vi "qSTE.vi"(0 "System no.":i32=1 min=1 max=4 step=1, 2 "Query axis":string, 5 "error in":errorcluster, 6 "Xo":i32, 7 "N":i32=100, 8 "Nmax":i32=1024) -> (14 "Step response":dbl[](array[numeric]) format="%.6f", 15 "Step size":dbl caption="Numeric" format="%.6f", 19 "error out":errorcluster)   [LabVIEW 2020]
doc: "GCS 1.0 controller: Returns N saved step response points. N must be less than or equal to Nmax. For large N values, communication timeout must be set long enough, otherwise a comm.error may occur.\nGCS 2.0 or higher: Returns STE settings. Use DRR? to read step response points back.\n\nC-843: VI reads step response points. Step size is not valid. Nmax = 32640.\n\nC-843.PM: VI reads step response points. Step size is not valid. Nmax = 32640.\n\nC-848: VI reads step response points. Step size is not valid. Nmax = 1024.\n\nC-866: VI reads step response points. Step size is not valid. Nmax = 32256.\n\nC-880: VI reads step response points. Step size is not valid. Nmax = 1024.\n\nE-517, E-518: VI reads STE settings. Step response is not valid. xo, N and Nmax are not valid.\n\nE-709: VI reads STE settings. Step response is not valid. xo, N and Nmax are not valid.\n\nE-710: VI reads step response points. Step size is not valid. Nmax = 8192.\n\nE-754: VI reads STE settings. Step response is not valid. xo, N and Nmax are not valid.\n\nE-755: VI reads STE settings. Step response, xo, N and Nmax are not valid.\n\nE-761: VI reads step response points. Step size is not valid. Nmax = 8192."
uses:
  Communication/Global1.vi
panel:
  # "GCS 1.0 controller: Returns N saved step response points. N must be \nless than or equal to Nmax. For large N values, communication timeout \nmust be set long enough, otherwise a comm.error may occur.\nGCS 2.0 or higher: Returns STE settings. Use DRR? to read impulse response \npoints back."
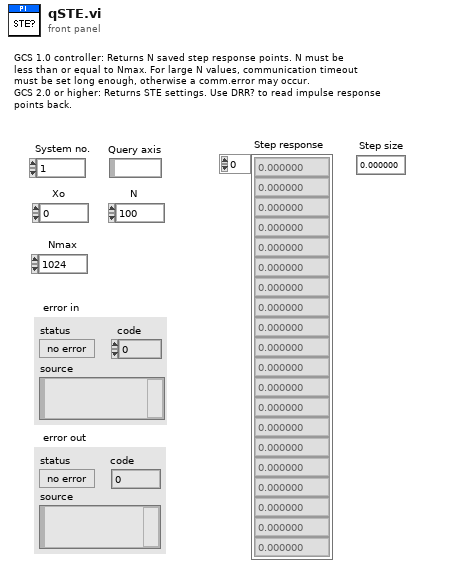
[diagram p1: front panel]
types:
  T1 = typedef "Syntax.ctl" = enum16{"GCS 1.0", "GCS 2.0", "GCS 3.0"}
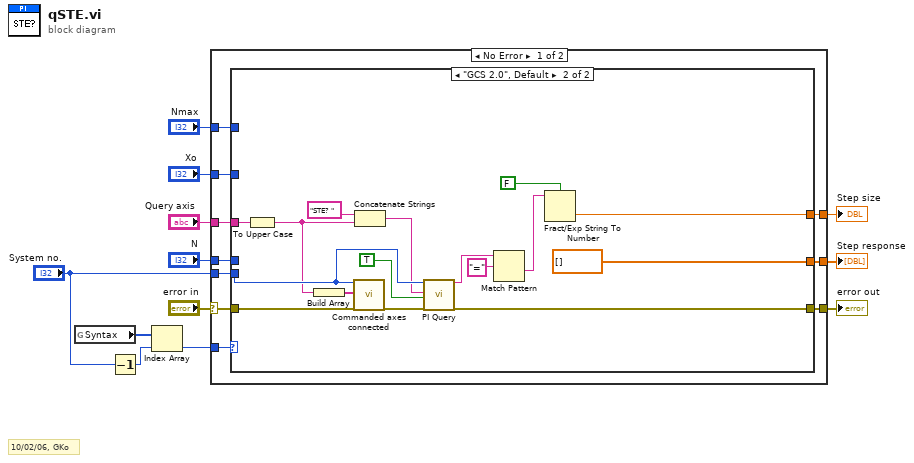
[diagram p0: block diagram]
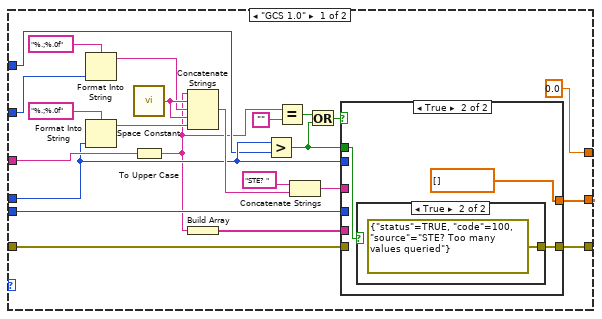
[diagram p2: hidden frame]
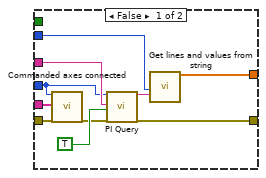
[diagram p3: hidden frame]
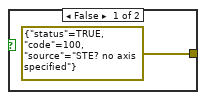
[diagram p4: hidden frame]
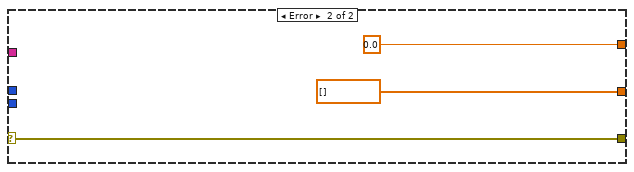
[diagram p5: hidden frame]
diagram:
  # "10/02/06, GKo"
  n1 = global read "Global1.vi" "Syntax"() -> (w5:T1[])
  n2 = Decrement(x="System no.") -> (x-1=w6:i32)
  n3 = Index Array(array=w5, index=w6) -> (element=w1:T1)
  n4 = case shown="No Error" "error in" {
    selector: "error in" -> [w14 w77]
    tunnel: "System no." -> [w22 _]
    tunnel: "Query axis" -> [w21 _]
    tunnel: [w20 w77] -> w11
    tunnel: [w19 dbl[] []] -> w10
    tunnel: "N" -> [w18 _]
    tunnel: "Xo" -> [w17 _]
    tunnel: "Nmax" -> [w16 _]
    tunnel: [w15 0.0] -> w3
    tunnel: w1 -> [w13 _]
    frame No Error {
      n5 = case shown="\"GCS 2.0\", Default" w13 {
        tunnel: w22 -> [w42 w73]
        tunnel: w21 -> [w40 w75]
        tunnel: [w37 w61] -> w20
        tunnel: [w36 dbl[] []] -> w19
        tunnel: w18 -> [w35 _]
        tunnel: w17 -> [w33 _]
        tunnel: w16 -> [w29 _]
        tunnel: w14 -> [w24 w69]
        tunnel: [0.0 w64] -> w15
        frame "GCS 1.0" {
          n6 = Format Into String(format string="%.;%.0f" ("Format String"), w33) -> (resulting string=w31:string)  [unwired: 2 in, 1 out]
          n7 = Format Into String(format string="%.;%.0f" ("Format String"), w35) -> (resulting string=w30:string)  [unwired: 2 in, 1 out]
          n8 = call <vilib>:"Space Constant.vi"() -> ("String"=w32:string)
          n9 = To Upper Case(1:w40) -> (0:w23:string)
          n10 = Concatenate Strings(w23, w32, w31, w32, w30) -> (w38:string)
          n11 = Build Array(w23) -> (w41:string[])
          n12 = Greater?(x=w35, y=w29) -> (0:w25:bool)
          n13 = Equal?(x=w23, y="" ("x")) -> (x = y?=w26:bool)
          n14 = Concatenate Strings("STE? ", w38) -> (w44:string)
          n15 = Or(x=w26, y=w25) -> (x .or. y?=w27:bool)
          n16 = case shown="True" w27 {
            tunnel: w44 -> [w54 _]
            tunnel: w42 -> [w52 _]
            tunnel: w41 -> [w51 _]
            tunnel: w24 -> [w53 _]
            tunnel: [w46 w57] -> w37
            tunnel: w35 -> [w49 _]
            tunnel: [w50 dbl[] [] ("Waveform points")] -> w36
            tunnel: w25 -> [_ w56]
            frame False {
              n17 = call "Commanded axes connected.vi"("System no."=w52, "Commanded axes"=w51, "error in"=w53) -> ("error out"=w48:errorcluster)  [unwired: 1 in, 15 out]
              n18 = call "PI Query.vi"("System no."=w52, "String to send"=w54, "Attach termination char.?"=TRUE ("Attach Linefeed?"), "error in"=w48) -> ("String read"=w47:string, "error out"=w46:errorcluster)  [unwired: 3 in, 11 out]
              n19 = call "Get lines and values from string.vi"("Array size"=w49, "Input string"=w47) -> ("Numerical values"=w50:dbl[])  [unwired: 17 out]
            }
            frame True {
              n20 = case shown="True" w56 {
                tunnel: [errorcluster {"status"=TRUE, "code"=100, "source"="STE? no axis specified"} ("error out") errorcluster {"status"=TRUE, "code"=100, "source"="STE? Too many values queried"} ("error out")] -> w57
                frame False {
                }
                frame True {
                }
              }
            }
          }
        }
        frame "GCS 2.0", Default {
          n21 = To Upper Case(1:w75) -> (0:w68:string)
          n22 = Build Array(w68) -> (w74:string[])
          n23 = call "Commanded axes connected.vi"("System no."=w73, "Commanded axes"=w74, "error in"=w69) -> ("error out"=w70:errorcluster)  [unwired: 1 in, 15 out]
          n24 = Concatenate Strings("STE? ", w68) -> (w71:string)
          n25 = call "PI Query.vi"("System no."=w73, "String to send"=w71, "Attach termination char.?"=TRUE ("Attach Linefeed?"), "error in"=w70) -> ("String read"=w62:string, "error out"=w61:errorcluster)  [unwired: 3 in, 11 out]
          n26 = Match Pattern(string=w62, regular expression="=") -> (after substring=w63:string)  [unwired: 4 out]
          n27 = Fract/Exp String To Number(use system decimal point (T)=FALSE, string=w63) -> (number=w64:dbl)  [unwired: 3 out]
        }
      }
    }
    frame Error {
    }
  }
  "error out" <- w11
  "Step response" <- w10
  "Step size" <- w3
